vi "rot1dArray.vi"(8 "error in (no error)":errorcluster, 10 "Rot Mat":dbl[][](array[numeric]), 11 "1D Array":dbl[](array[numeric])) -> (0 "error out":errorcluster, 3 "Rotated 1D Array":dbl[](array[numeric]))   [LabVIEW 2016]
doc: "Rotate the 1D array based on the rotation matrix."
uses:
  <vilib>/Analysis/baseanly.llb/Real A x B.vi
  <vilib>/Analysis/Matrix/Numeric/Conversions/Array To Matrix - RA2.vi
  <vilib>/Analysis/Matrix/Numeric/Conversions/Matrix To Array - RM.vi
  <vilib>/Analysis/Matrix/NI_Matrix.lvlib
  <vilib>/Analysis/NI_AALBase.lvlib
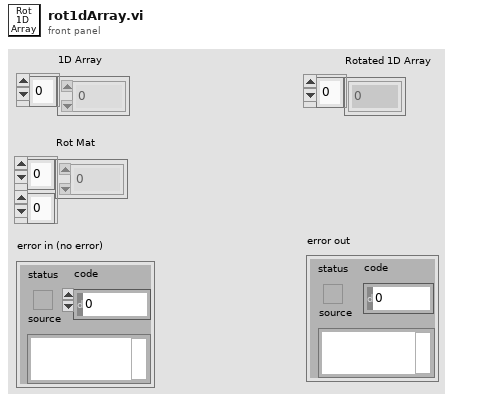
[diagram p1: front panel]
types:
  T1 = typedef "NI_Matrix.lvlib/RealMatrix.ctl" = dbl[][]
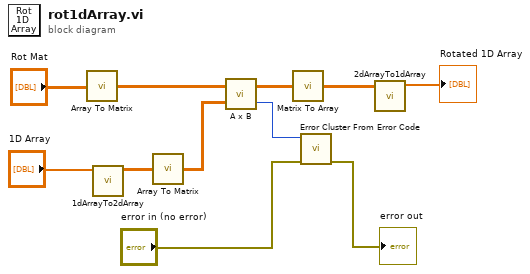
[diagram p0: block diagram]
diagram:
  n1 = call-poly <vilib>:"Array To Matrix.vi"("Real 2D Array"="Rot Mat") -> ("Real Matrix"=w8:T1)
  n2 = call "1dArrayTo2dArray.vi"("1D Array"="1D Array") -> ("2D Array"=w10:dbl[][])  [unwired: 10 in]
  n3 = call-poly <vilib>:"Array To Matrix.vi"("Real 2D Array"=w10) -> ("Real Matrix"=w7:T1)
  n4 = call-poly <vilib>:"A x B.vi"("B"=w7, "A"=w8) -> ("error"=w6:i32, "A x B"=w3:T1)
  n5 = call-poly <vilib>:"Matrix To Array.vi"("Real Matrix"=w3) -> ("Real 2D Array"=w2:dbl[][])
  n6 = call <vilib>:"Error Cluster From Error Code.vi"("error in (no error)"="error in (no error)", "error code (0)"=w6) -> ("error out"=→"error out":errorcluster)  [unwired: 7 in]
  n7 = call "2dArrayTo1dArray.vi"("2D Array"=w2) -> ("1D Array"=→"Rotated 1D Array":dbl[])  [unwired: 10 in]
